vi "工控机配置.vi"() -> ()   [LabVIEW 2013]
uses:
  <vilib>/Utility/config.llb/Write Key (I32).vi
  <vilib>/Utility/config.llb/Read Key (I32).vi
  <vilib>/Utility/config.llb/NI_LVConfig.lvlib
panel:
  out "Array":dbl[](array[numeric])
  in  "电气":T1(radio)=enum."ai0"
  in  "油压2":T1(radio)=enum."ai0"
  in  "退出":bool
  in  "油压1":T1(radio)=enum."ai0"
  in  "行程":T1(radio)=enum."ai0"
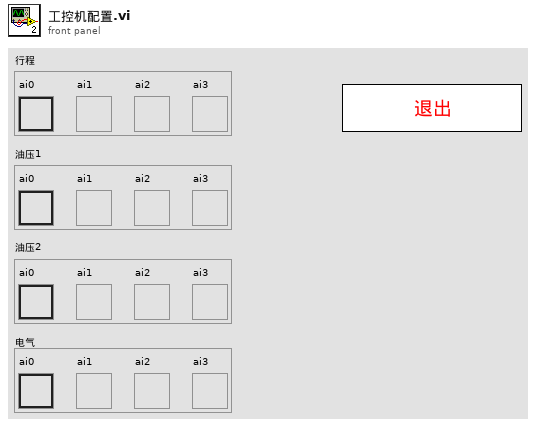
[diagram p1: front panel]
types:
  T1 = enum32{"No Selection", "ai0", "ai1", "ai2", "ai3"}
  T2 = typedef "NI_LVConfig.lvlib/Config Data RefNum.ctl" = refnum<k1>
  T3 = enum32{"No Selection", "ai0", "ai1", "ai2", "ai3"}[]
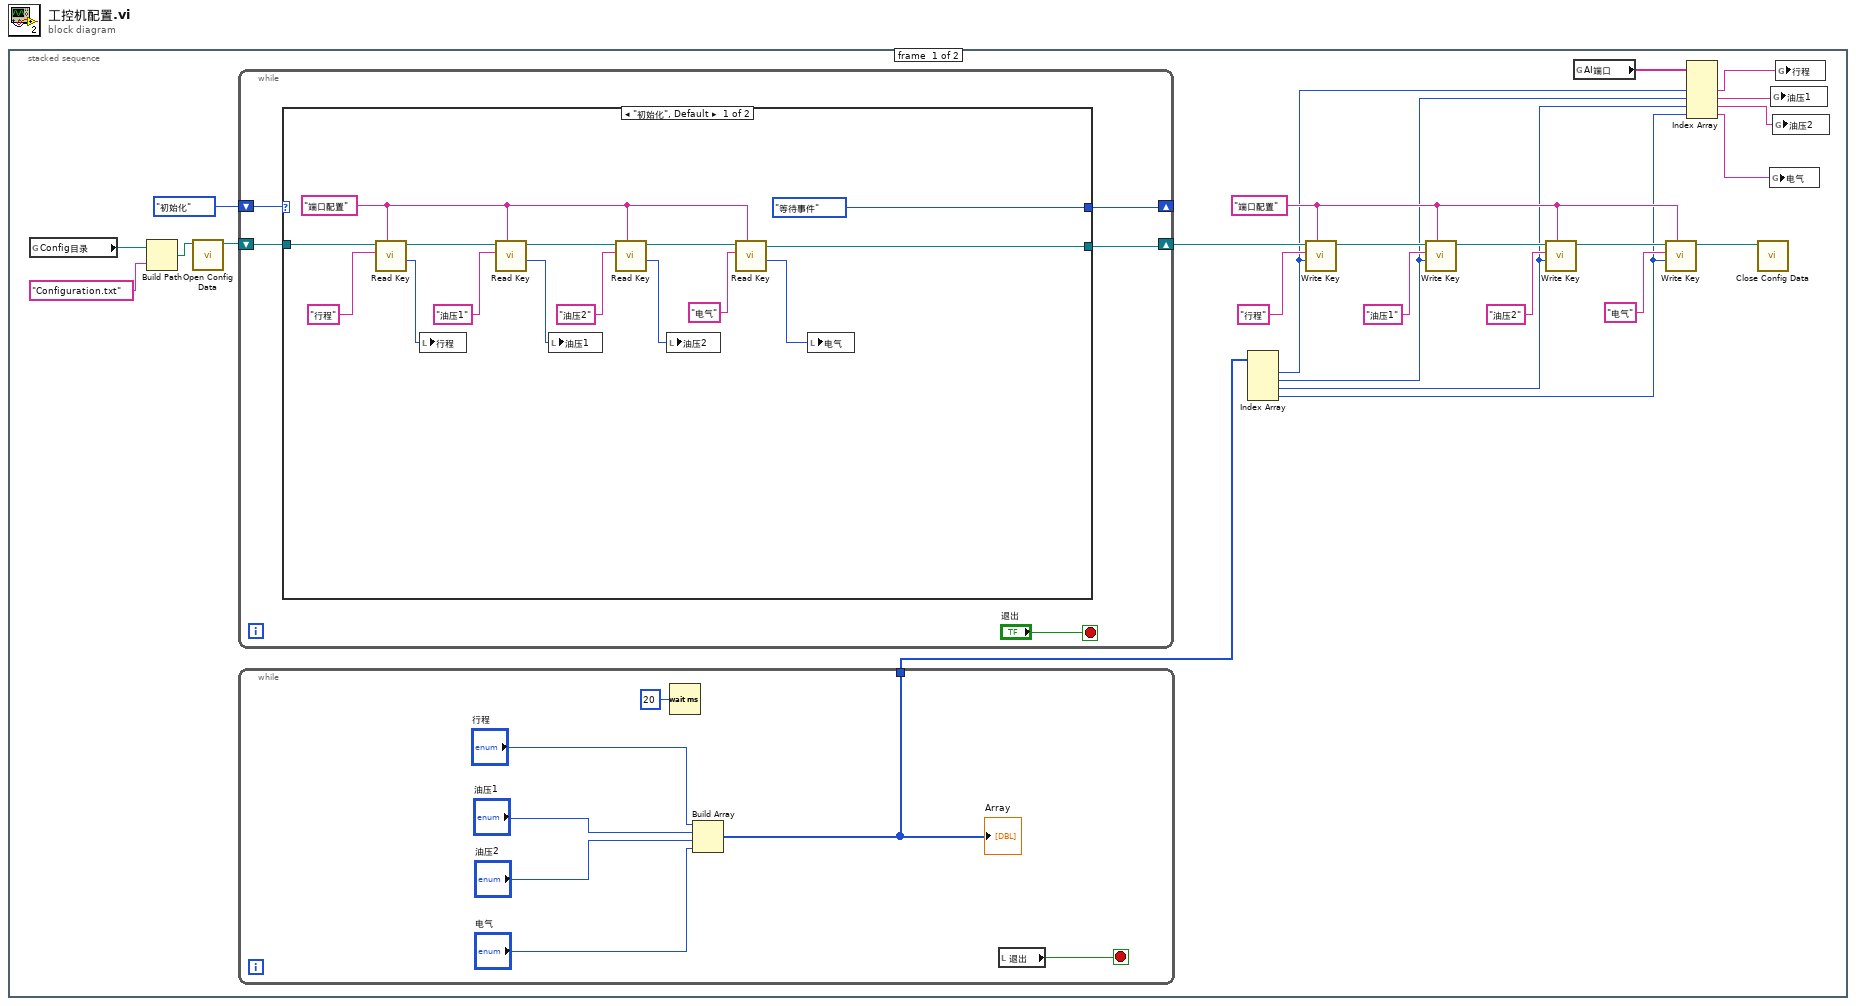
[diagram p0: block diagram]
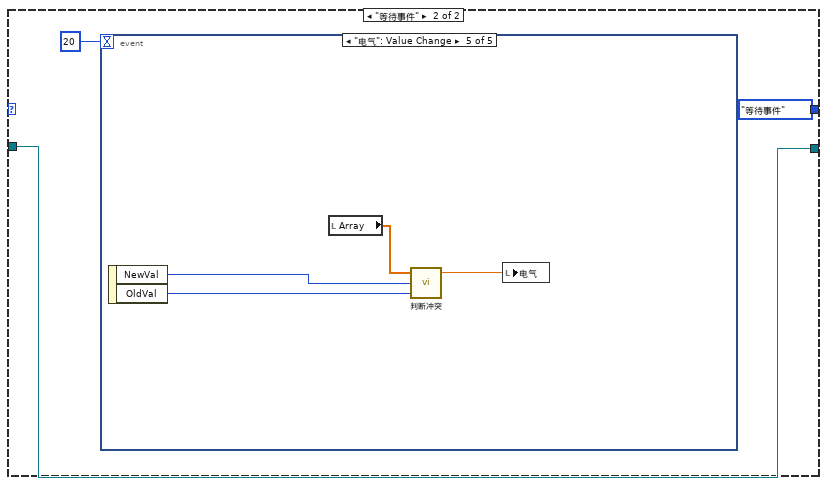
[diagram p2: hidden frame]
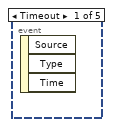
[diagram p3: hidden frame]
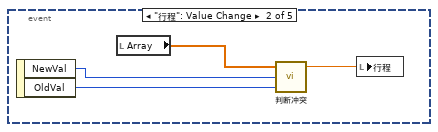
[diagram p4: hidden frame]
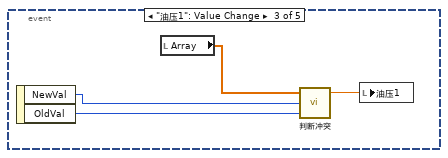
[diagram p5: hidden frame]
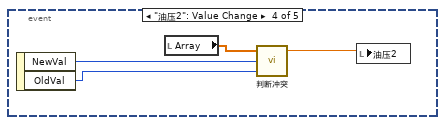
[diagram p6: hidden frame]
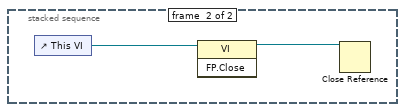
[diagram p7: hidden frame]
diagram:
  n1 = stacked-sequence {
    frame #0 {
      w18 = "端口配置" ("Section")
      n2 = global read "Config目录.vi" "Config目录"() -> (w24:path)
      n3 = Build Path(base path=w24, name or relative path="Configuration.txt") -> (appended path=w14:path)
      n4 = call <vilib>:"Open Config Data.vi"("configuration file path"=w14) -> ("refnum"=w13:T2)  [unwired: 8 in, 2 out]
      n5 = while {
        shift-right: [w35] -> _
        shift-left: enum16{"初始化", "等待事件"}."初始化" -> [w37]
        shift-right: [w33] -> w12
        shift-left: w13 -> [w34]
        stop <- "退出" stop-if-true
        n6 = case shown="\"初始化\", Default" w37 {
          tunnel: [enum16{"初始化", "等待事件"}."等待事件" enum16{"初始化", "等待事件"}."等待事件"] -> w35
          tunnel: w34 -> [w38 w53]
          tunnel: [w39 w53] -> w33
          frame "初始化", Default {
            w47 = "端口配置" ("Section")
            n7 = call-poly <vilib>:"Read Key.vi"("section"=w47, "key"="行程" ("Key"), "refnum"=w38) -> ("value"=w51:i32, "refnum out"=w50:T2)  [unwired: 5 in, 2 out]
            n8 = local write "行程"(w51) -> ()
            n9 = call-poly <vilib>:"Read Key.vi"("section"=w47, "key"="油压1" ("Key"), "refnum"=w50) -> ("value"=w45:i32, "refnum out"=w49:T2)  [unwired: 5 in, 2 out]
            n10 = local write "油压1"(w45) -> ()
            n11 = call-poly <vilib>:"Read Key.vi"("section"=w47, "key"="油压2" ("Key"), "refnum"=w49) -> ("value"=w40:i32, "refnum out"=w48:T2)  [unwired: 5 in, 2 out]
            n12 = local write "油压2"(w40) -> ()
            n13 = call-poly <vilib>:"Read Key.vi"("section"=w47, "key"="电气" ("Key"), "refnum"=w48) -> ("value"=w41:i32, "refnum out"=w39:T2)  [unwired: 5 in, 2 out]
            n14 = local write "电气"(w41) -> ()
          }
          frame "等待事件" {
            n15 = event shown="[4] \"电气\": Value Change" {
              selector: _ -> [_ _ _ _ _]
              dyn-events: _ -> [_ _ _ _ _]
              timeout: 20 -> [_ _ _ _ _]
              event Timeout {
                n16 = event-data() -> ()  [unwired: 1 in, 3 out]
              }
              event "行程": Value Change {
                n17 = event-data() -> ("NewVal"=w58:T1, "OldVal"=w57:T1)  [unwired: 1 in]
                n18 = local read "Array"() -> (w59:dbl[])
                n19 = call "判断冲突.vi"("OldVal"=w57, "NewVal"=w58, "Array"=w59) -> ("OutVal"=w56:dbl)  [unwired: 2 in]
                n20 = local write "行程"(w56) -> ()
              }
              event "油压1": Value Change {
                n21 = event-data() -> ("NewVal"=w62:T1, "OldVal"=w63:T1)  [unwired: 1 in]
                n22 = local read "Array"() -> (w61:dbl[])
                n23 = call "判断冲突.vi"("OldVal"=w63, "NewVal"=w62, "Array"=w61) -> ("OutVal"=w60:dbl)  [unwired: 2 in]
                n24 = local write "油压1"(w60) -> ()
              }
              event "油压2": Value Change {
                n25 = event-data() -> ("NewVal"=w64:T1, "OldVal"=w65:T1)  [unwired: 1 in]
                n26 = local read "Array"() -> (w66:dbl[])
                n27 = call "判断冲突.vi"("OldVal"=w65, "NewVal"=w64, "Array"=w66) -> ("OutVal"=w67:dbl)  [unwired: 2 in]
                n28 = local write "油压2"(w67) -> ()
              }
              event "电气": Value Change {
                n29 = event-data() -> ("NewVal"=w69:T1, "OldVal"=w70:T1)  [unwired: 1 in]
                n30 = local read "Array"() -> (w68:dbl[])
                n31 = call "判断冲突.vi"("OldVal"=w70, "NewVal"=w69, "Array"=w68) -> ("OutVal"=w71:dbl)  [unwired: 2 in]
                n32 = local write "电气"(w71) -> ()
              }
            }
          }
        }
      }
      n33 = while {
        tunnel: [w26] -> w10
        stop <- w27 stop-if-true
        n34 = Wait (ms)(milliseconds to wait=u32 20) -> ()  [unwired: 1 out]
        n35 = Build Array("行程", "油压1", "油压2", "电气") -> (w26:T3)
        "Array" <- w26
        n36 = local read "退出"() -> (w27:bool)
      }
      n37 = Index Array(array=w10) -> (element #1=w6:T1, element #2=w5:T1, element #3=w4:T1, element #4=w3:T1)  [unwired: 4 in]
      n38 = call-poly <vilib>:"Write Key.vi"("section"=w18, "value"=w6, "key"="行程" ("Key"), "refnum"=w12) -> ("refnum out"=w21:T2)  [unwired: 5 in, 2 out]
      n39 = call-poly <vilib>:"Write Key.vi"("section"=w18, "value"=w5, "key"="油压1" ("Key"), "refnum"=w21) -> ("refnum out"=w20:T2)  [unwired: 5 in, 2 out]
      n40 = call-poly <vilib>:"Write Key.vi"("section"=w18, "value"=w4, "key"="油压2" ("Key"), "refnum"=w20) -> ("refnum out"=w19:T2)  [unwired: 5 in, 2 out]
      n41 = global read "AI端口.vi" "AI端口"() -> (w9:tag[])
      n42 = call-poly <vilib>:"Write Key.vi"("section"=w18, "value"=w3, "key"="电气" ("Key"), "refnum"=w19) -> ("refnum out"=w11:T2)  [unwired: 5 in, 2 out]
      n43 = Index Array(array=w9, index #2=w6, index #3=w5, index #4=w4, index #5=w3) -> (element #2=w8:tag, element #3=w7:tag, element #4=w2:tag, element #5=w1:tag)  [unwired: 1 in, 1 out]
      n44 = call <vilib>:"Close Config Data.vi"("refnum"=w11) -> ()  [unwired: 9 in, 2 out]
      n45 = global write "AI端口_电气.vi" "电气"(w1) -> ()
      n46 = global write "AI端口_油压1.vi" "油压1"(w7) -> ()
      n47 = global write "AI端口_油压2.vi" "油压2"(w2) -> ()
      n48 = global write "AI端口_行程.vi" "行程"(w8) -> ()
    }
    frame #1 {
      n49 = control-ref of="This VI"() -> (w72:refnum<vi>)
      n50 = invoke class="VI" method="FP.Close"(reference=w72) -> (reference out=w73:refnum<vi>)  [unwired: 2 in, 2 out]
      n51 = Close Reference(reference=w73) -> ()  [unwired: 1 in, 1 out]
    }
  }
